vi "FPGANic-Tester.vi"() -> ()   [LabVIEW 2017]
uses:
  Source.Machine.Settings.ctl
  FPGANic.Events.ctl
  <vilib>/FPGAPlugInAG/PXIe-6592R/niLvFpga_Open_PXIe-6592R.vi
  <vilib>/rvi/interface/common/dynamic/niFpgaDynamicAddResources.vi
  FPGANic.Globals.vi
  <vilib>/Utility/error.llb/Error Cluster From Error Code.vi
  <vilib>/rvi/errors/niLvFpgaAdjustHostInterfaceError.vi
  <vilib>/FPGAPlugInAG/Dynamic/niLvFpga_Close_Dynamic.vi
  <vilib>/rvi/interface/nirviOpenFPGA/nirviOpenFPGA.xnode
  FPGA Bitfiles/FPGANic-Top.lvbitx
  <vilib>/rvi/interface/nirviMethod/nirviMethod.xnode
  <vilib>/rvi/interface/nirviReadWriteControl/nirviReadWriteControl.xnode
  <vilib>/rvi/interface/nirviCloseFPGA/nirviCloseFPGA.xnode
  <vilib>/FPGAPlugInAG/Dynamic/niLvFpga_ReadFifo_Dynamic.vi
  <vilib>/rvi/errors/niLvFpgaMergeErrorWithErrorCode.vi
  <vilib>/FPGAPlugInAG/Dynamic/niLvFpga_WriteFifo_Dynamic.vi
  NiFpgaLv.dll
  <vilib>/rvi/interface/Simulation/niFpgaSimulationCallBeginRW.vi
panel:
  in  "Read Probes":bool
  in  "Read Debug FIFOs":bool
  in  "Tab Control":T1(tab)
  in  "Ethernet II Params":T2={"Destination MAC"=[0, 2, 201, 85, 8, 68], "Source MAC"=[0, 1, 2, 3, 4, 5], "EtherType"=2048} {"Destination MAC" format="%.0x"; "Source MAC" format="%.02x"; "EtherType" format="%.0x"}
  in  "IPv4 Params":T3={"Destination IP"=[10, 0, 1, 100], "Source IP"=[10, 0, 1, 101], "Protocol"=17}
  in  "UDP Params":T4={"Source Port"=35312, "Destination Port"=35312, "Payload"="ABCD"}
  in  "MAC & IP":T5={"MAC Address"=[0, 1, 2, 3, 4, 5], "IP Address"=[10, 0, 1, 101]} {"MAC Address" format="%.0x"}
  out "Write Probe 2":u64[](array[numeric]) format="%.0x"
  out "Write Probe 1":u64[](array[numeric]) format="%.0x"
  out "Read Probe":u64[](array[numeric]) format="%.0x"
  out "Debug FIFO 2":u32[](array[numeric]) format="%.0x"
  out "Debug FIFO 1":u32[](array[numeric]) format="%.0x"
  out "UDP Payload":u8[](array[numeric]) format="%.0x"
  in  "Clear Debug FIFOS?":bool=TRUE
  in  "AXI_STR_RXD_3_tkeep":u8=15
  out "GPIO #1 out":u32 format="%.0x"
  in  "GPIO #2 in":u32 format="%.0x"
  in  "GPIO #1 in":u32=4 format="%.0x"
  out "GPIO #2 out":u32
  out "sPort0_Power_Good":bool
  out "signal_detect_Port0":bool
  out "aBlockLockPort0":bool
  in  "Read/Write GPIO":bool
  out "error out":errorcluster
  out "Status":string
  in  "error in":errorcluster
  in  "Exit":bool
  in  "Transmit Packet":bool
  in  "Read Packet":bool
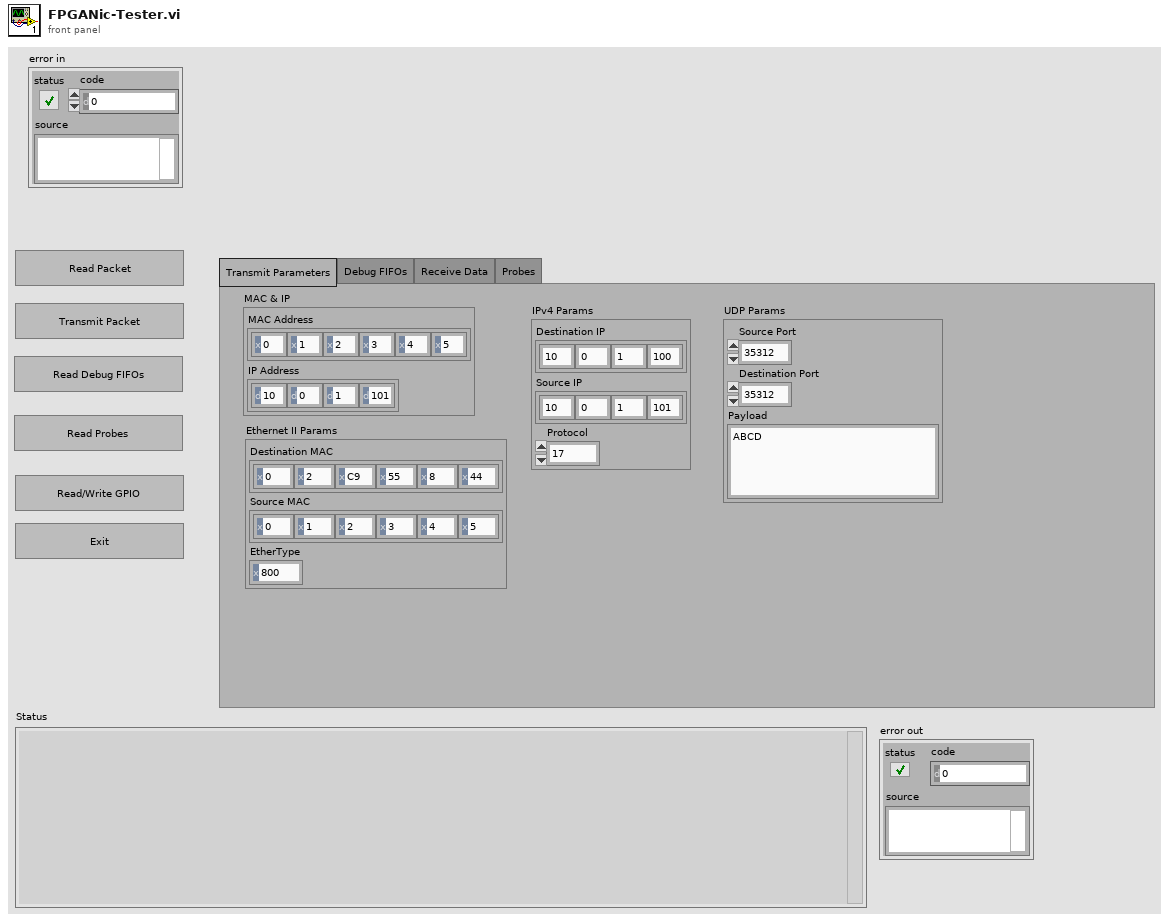
[diagram p1: front panel]
types:
  T1 = enum32{"Transmit Parameters", "Debug FIFOs", "Receive Data", "Probes"}
  T2 = cluster{"Destination MAC":u8[], "Source MAC":u8[], "EtherType":u16}
  T3 = cluster{"Destination IP":u8[], "Source IP":u8[], "Protocol":u8}
  T4 = cluster{"Source Port":u16, "Destination Port":u16, "Payload":string}
  T5 = typedef "Source.Machine.Settings.ctl" = cluster{"MAC Address":u8[], "IP Address":u8[]}
  T6 = typedef "FPGANic.Events.ctl" = enum16{"Open FPGA", "Close FPGA", "Reset UI", "Read Packet", "Transmit Packet", "Read Debug FIFOs", "Read Probes", "Read/Write GPIO"}
  T7 = cluster{"Read Probe":u64[], "Write Probe 1":u64[], "Write Probe 2":u64[], "Debug FIFO 1":u32[], "Debug FIFO 2":u32[]}
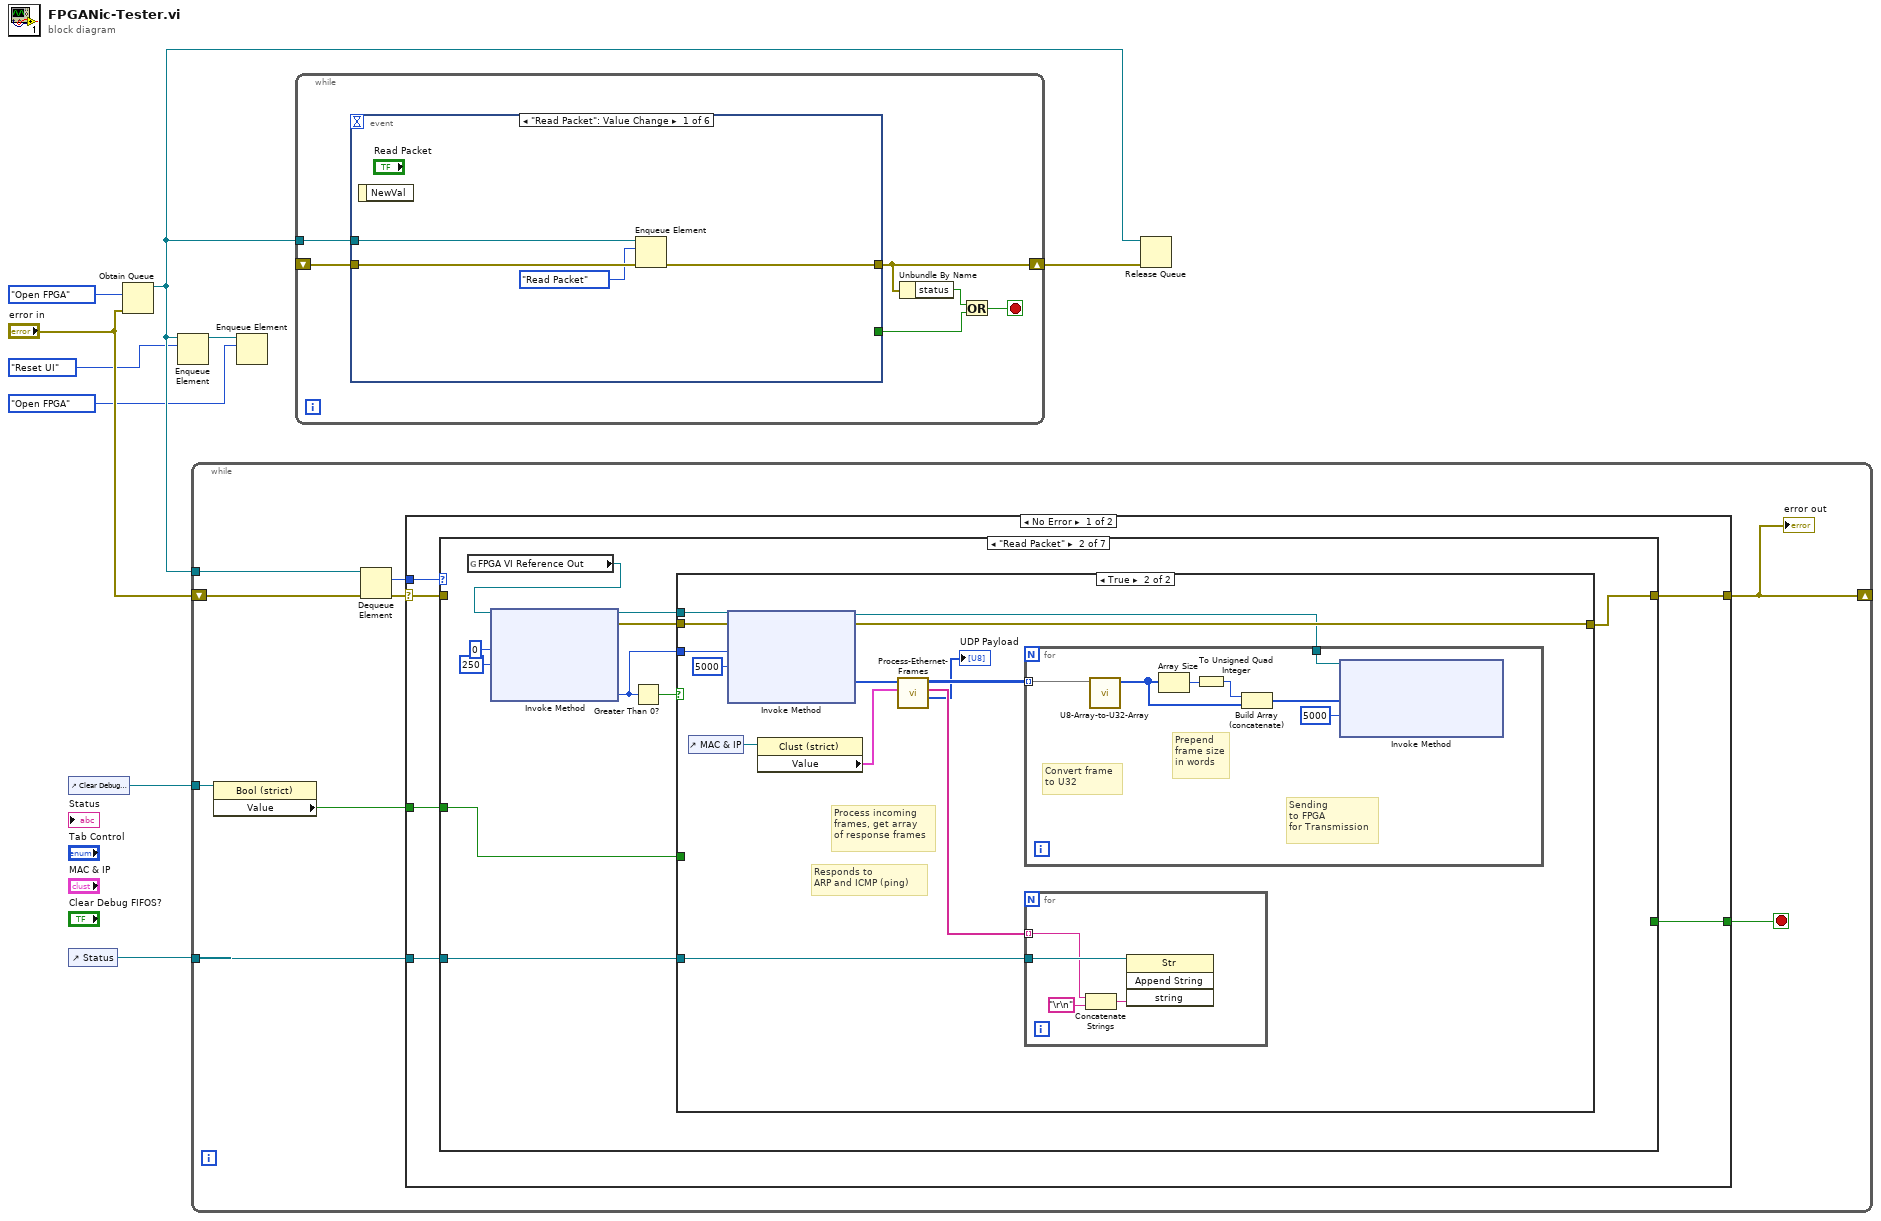
[diagram p0: block diagram]
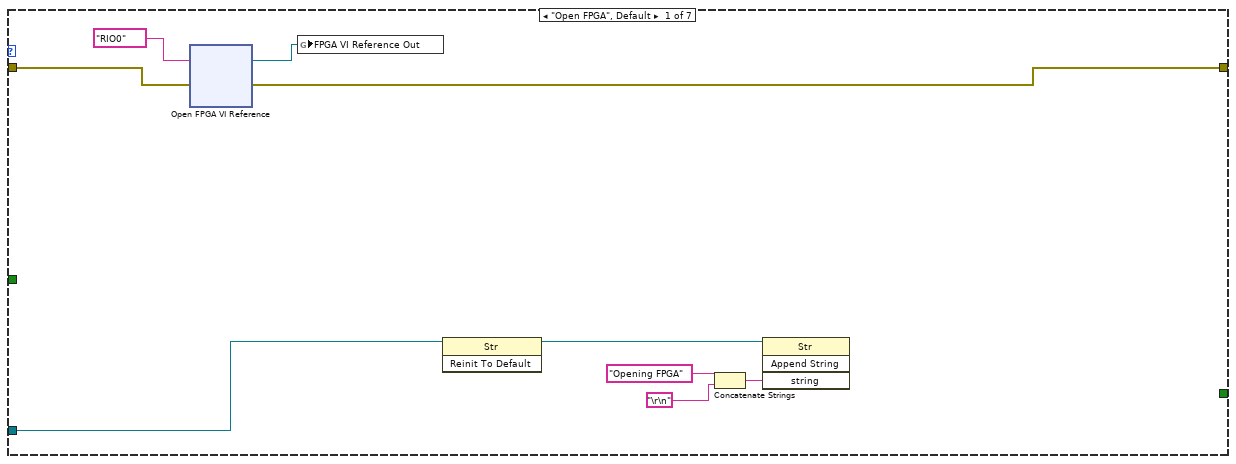
[diagram p2: hidden frame]
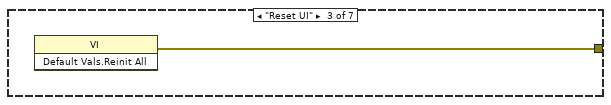
[diagram p4: hidden frame]
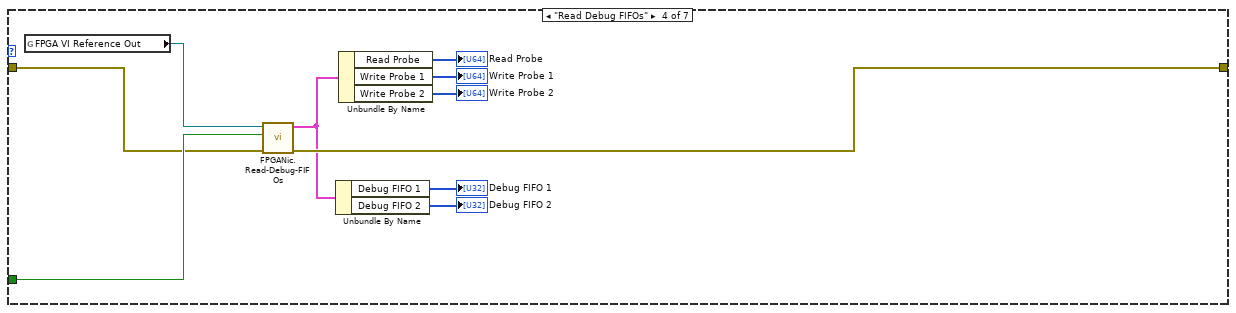
[diagram p5: hidden frame]
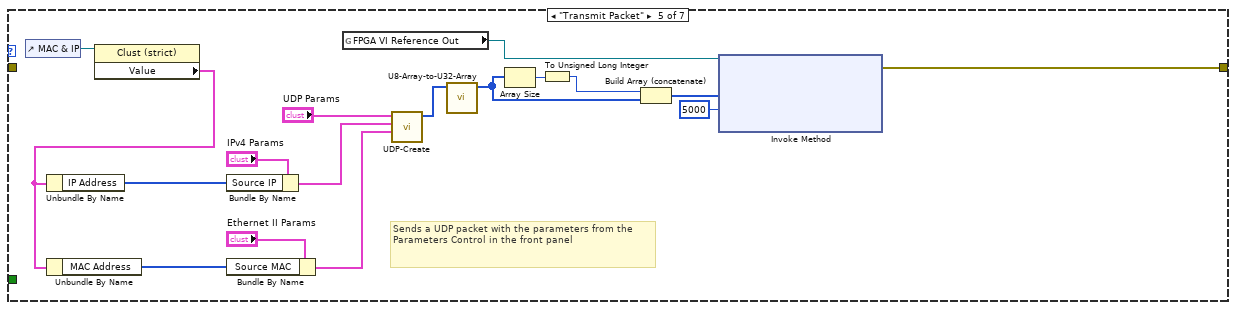
[diagram p6: hidden frame]
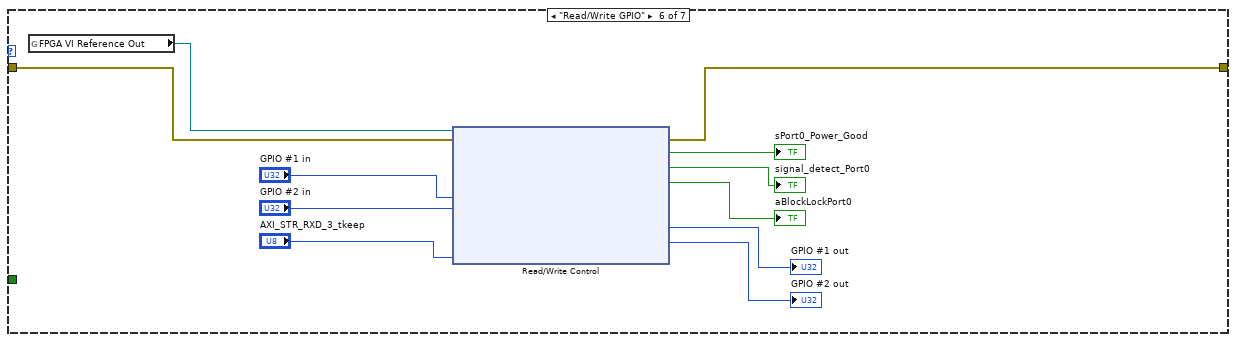
[diagram p7: hidden frame]
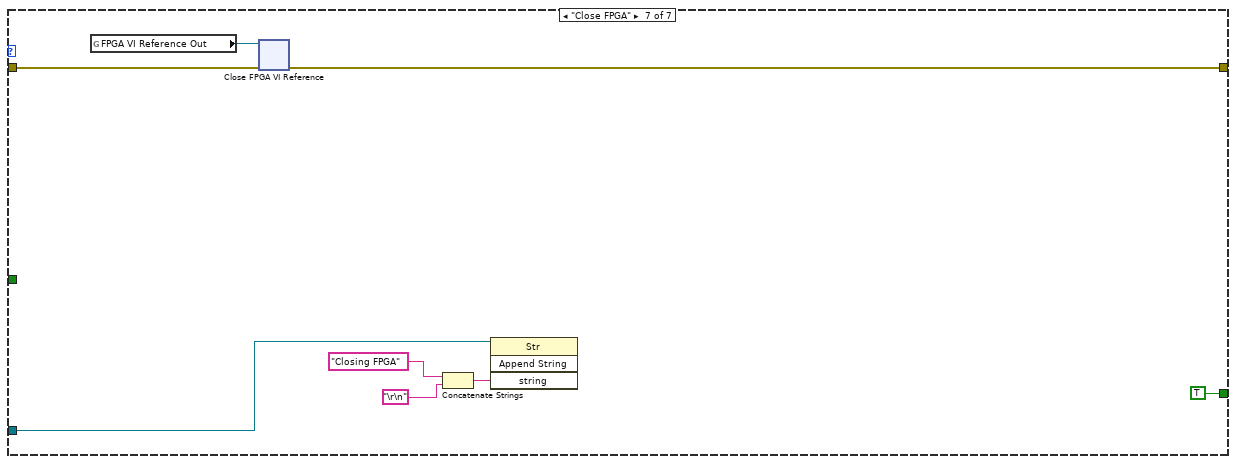
[diagram p8: hidden frame]
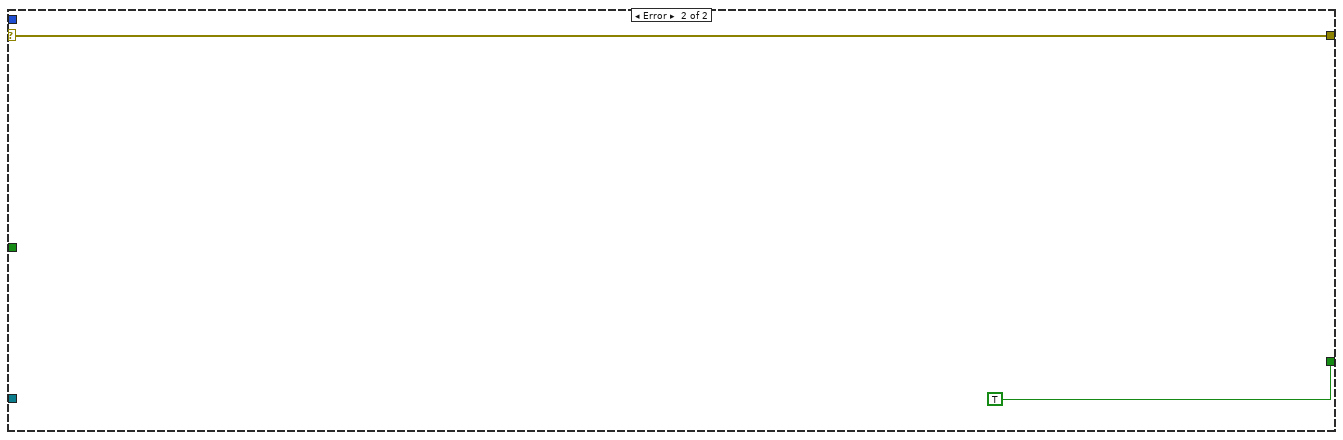
[diagram p9: hidden frame]
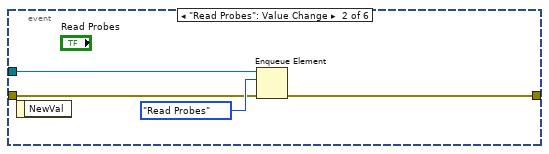
[diagram p10: hidden frame]
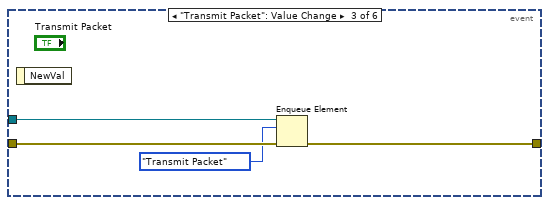
[diagram p11: hidden frame]
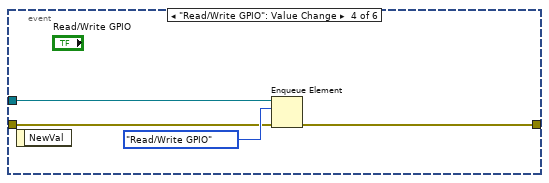
[diagram p12: hidden frame]
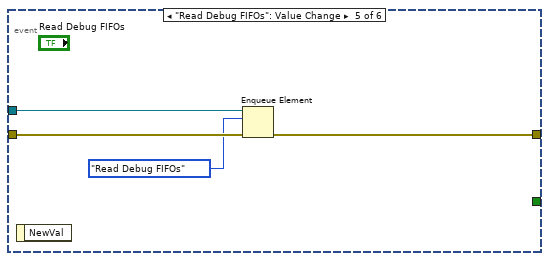
[diagram p13: hidden frame]
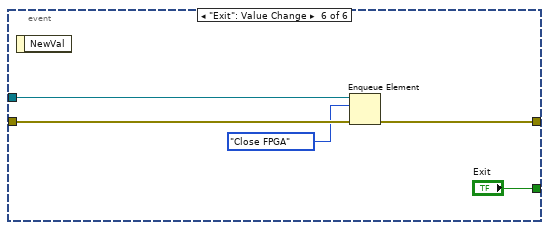
[diagram p14: hidden frame]
diagram:
  n1 = control-ref of="Clear Debug FIFOS?"() -> (w4:refnum<vi>)
  n2 = control-ref of="Status"() -> (w5:refnum<vi>)
  n3 = Obtain Queue(element data type=FPGANic.Events."Open FPGA" ("Enum"), error in (no error)="error in") -> (queue out=w7:refnum<queue>)  [unwired: 3 in, 2 out]
  n4 = Enqueue Element(queue=w7, element=FPGANic.Events."Reset UI" ("Enum")) -> (queue out=w3:refnum<queue>)  [unwired: 2 in, 2 out]
  n5 = while {
    tunnel: w7 -> [w18]
    shift-right: [w13] -> _
    shift-left: "error in" -> [w14]
    tunnel: w5 -> [w12]
    tunnel: w4 -> [w11]
    stop <- w15 stop-if-true
    n6 = property class="Bool (strict)"(reference=w11) -> ("Value"=w10:bool)  [unwired: 1 in, 2 out]
    n7 = Dequeue Element(queue=w18, error in (no error)=w14) -> (element=w16:T6, error out=w17:errorcluster)  [unwired: 1 in, 2 out]
    n8 = case shown="No Error" w17 {
      selector: w17 -> [w19 w116]
      tunnel: w16 -> [w24 _]
      tunnel: [w23 TRUE] -> w15
      tunnel: [w22 w116] -> w13
      tunnel: w12 -> [w21 _]
      tunnel: w10 -> [w20 _]
      frame No Error {
        n9 = case shown="\"Read Packet\"" w24 {
          tunnel: [_ _ _ _ _ _ TRUE] -> w23
          tunnel: [w33 w38 w69 w77 w94 w99 w114] -> w22
          tunnel: w21 -> [w29 w34 _ _ _ _ w110]
          tunnel: w20 -> [_ w36 _ w78 _ _ _]
          tunnel: w19 -> [w26 _ _ w76 _ w97 w108]
          frame "Open FPGA", Default {
            n10 = xnode "Open FPGA VI Reference"("error in"=w26, "resource name"=tag "RIO0") -> ("FPGA VI Reference Out"=w25:refnum<k20>, "error out"=w33:errorcluster)
            n11 = global write "FPGANic.Globals.vi" "FPGA VI Reference Out"(w25) -> ()
            n12 = invoke class="Str" method="Reinit To Default"(reference=w29) -> (reference out=w28:refnum<vi>)  [unwired: 2 in, 2 out]
            n13 = Concatenate Strings("Opening FPGA" ("string"), "\r\n") -> (w32:string)
            n14 = invoke class="Str" method="Append String"(reference=w28, "string"=w32) -> ()  [unwired: 2 in, 4 out]
          }
          frame "Read Packet" {
            n15 = global read "FPGANic.Globals.vi" "FPGA VI Reference Out"() -> (w35:refnum<k20>)
            n16 = xnode "Invoke Method"("FPGA VI Reference In"=w35, "Number of Elements"=u32 0, "Timeout (ms)"=250) -> ("FPGA VI Reference Out"=w40:refnum<k20>, "error out"=w39:errorcluster, "Elements Remaining"=w37:u32)  [unwired: 1 in, 1 out]
            n17 = Greater Than 0?(x=w37) -> (x > 0?=w41:bool)
            n18 = case shown="True" w41 {
              tunnel: w40 -> [_ w56]
              tunnel: w39 -> [w44 w55]
              tunnel: [w44 w53] -> w38
              tunnel: w37 -> [_ w54]
              tunnel: w36 -> [_ _]
              tunnel: w34 -> [_ w47]
              frame False {
              }
              frame True {
                # "Responds to\nARP and ICMP (ping)"
                # "Process incoming\nframes, get array\nof response frames"
                n19 = control-ref of="MAC & IP"() -> (w50:refnum<vi>)
                n20 = xnode "Invoke Method"("FPGA VI Reference In"=w56, "error in"=w55, "Number of Elements"=w54, "Timeout (ms)"=5000) -> ("FPGA VI Reference Out"=w48:refnum<k20>, "error out"=w53:errorcluster, "Data"=w52:u64[])  [unwired: 1 out]
                n21 = property class="Clust (strict)"(reference=w50) -> ("Value"=w49:T5)  [unwired: 1 in, 2 out]
                n22 = call "Process-Ethernet-Frames.vi"("Source Machine\nSettings"=w49, "Raw Data\nStream"=w52) -> ("UDP Payload"=→"UDP Payload":u8[], "Messages"=w46:string[], "Frames to send"=w51:u8[][])  [unwired: 7 in]
                n23 = for {
                  tunnel: w51 -> [w68] mode=indexing
                  tunnel: w48 -> [w62]
                  # "Prepend\nframe size\nin words"
                  # "Sending\nto FPGA\nfor Transmission"
                  # "Convert frame\nto U32"
                  n24 = call "U8-Array-to-U32-Array.vi"("Frame U8[] in"=w68) -> ("Frame U32[] out"=w63:u32[])  [unwired: 10 in]
                  n25 = Array Size(array=w63) -> (size(s)=w67:i32)
                  n26 = To Unsigned Quad Integer(1:w67) -> (0:w66:u64)
                  n27 = Build Array (concatenate)(w66, w63) -> (w65:u64[])
                  n28 = xnode "Invoke Method"("FPGA VI Reference In"=w62, "Data"=w65, "Timeout (ms)"=5000) -> ()  [unwired: 1 in, 3 out]
                }
                n29 = for {
                  tunnel: w47 -> [w59]
                  tunnel: w46 -> [w58] mode=indexing
                  n30 = Concatenate Strings(w58, "\r\n") -> (w61:string)
                  n31 = invoke class="Str" method="Append String"(reference=w59, "string"=w61) -> ()  [unwired: 2 in, 4 out]
                }
              }
            }
          }
          frame "Reset UI" {
            n32 = invoke class="VI" method="Default Vals.Reinit All"() -> (error out=w69:errorcluster)  [unwired: 3 in, 2 out]
          }
          frame "Read Debug FIFOs" {
            n33 = global read "FPGANic.Globals.vi" "FPGA VI Reference Out"() -> (w79:refnum<k20>)
            n34 = call "FPGANic.Read-Debug-FIFOs.vi"("error in"=w76, "Value"=w78, "FPGA VI Reference Out"=w79) -> ("error out"=w77:errorcluster, "Debug Data"=w72:T7)  [unwired: 7 in]
            n35 = Unbundle By Name(w72) -> ("Debug FIFO 1"=→"Debug FIFO 1":u32[], "Debug FIFO 2"=→"Debug FIFO 2":u32[])
            n36 = Unbundle By Name(w72) -> ("Read Probe"=→"Read Probe":u64[], "Write Probe 1"=→"Write Probe 1":u64[], "Write Probe 2"=→"Write Probe 2":u64[])
          }
          frame "Transmit Packet" {
            # "Sends a UDP packet with the parameters from the\nParameters Control in the front panel"
            n37 = control-ref of="MAC & IP"() -> (w83:refnum<vi>)
            n38 = property class="Clust (strict)"(reference=w83) -> ("Value"=w81:T5)  [unwired: 1 in, 2 out]
            n39 = Unbundle By Name(w81) -> ("IP Address"=w82:u8[])
            n40 = Unbundle By Name(w81) -> ("MAC Address"=w80:u8[])
            n41 = Bundle By Name(cluster="IPv4 Params", "Source IP"=w82) -> (w84:T3)
            n42 = Bundle By Name(cluster="Ethernet II Params", "Source MAC"=w80) -> (w85:T2)
            n43 = global read "FPGANic.Globals.vi" "FPGA VI Reference Out"() -> (w93:refnum<k20>)
            n44 = call "UDP-Create.vi"("Ethernet II Params"=w85, "IPv4 Params"=w84, "UDP Params"="UDP Params") -> ("Ethernet Frame"=w92:u8[])  [unwired: 6 in, 2 out]
            n45 = call "U8-Array-to-U32-Array.vi"("Frame U8[] in"=w92) -> ("Frame U32[] out"=w89:u32[])  [unwired: 10 in]
            n46 = Array Size(array=w89) -> (size(s)=w91:i32)
            n47 = To Unsigned Long Integer(number=w91) -> (unsigned 32bit integer=w90:u32)
            n48 = Build Array (concatenate)(w90, w89) -> (w88:u32[])
            n49 = xnode "Invoke Method"("FPGA VI Reference In"=w93, "Data"=w88, "Timeout (ms)"=5000) -> ("error out"=w94:errorcluster)  [unwired: 1 in, 2 out]
          }
          frame "Read/Write GPIO" {
            n50 = global read "FPGANic.Globals.vi" "FPGA VI Reference Out"() -> (w98:refnum<k20>)
            n51 = xnode "Read/Write Control"("FPGA VI Reference In"=w98, "error in"=w97, "GPIO #1 in"="GPIO #1 in", "GPIO #2 in"="GPIO #2 in", "d_microblaze_i\\AXI_STR_RXD_3_tkeep"="AXI_STR_RXD_3_tkeep") -> ("error out"=w99:errorcluster, "sPort0_Power_Good"=→"sPort0_Power_Good":bool, "signal_detect_Port0"=→"signal_detect_Port0":bool, "aBlockLockPort0"=→"aBlockLockPort0":bool, "GPIO #1 out"=→"GPIO #1 out":u32, "GPIO #2 out"=→"GPIO #2 out":u32)  [unwired: 1 out]
          }
          frame "Close FPGA" {
            n52 = global read "FPGANic.Globals.vi" "FPGA VI Reference Out"() -> (w109:refnum<k20>)
            n53 = xnode "Close FPGA VI Reference"("FPGA VI Reference In"=w109, "error in"=w108) -> ("error out"=w114:errorcluster)
            n54 = Concatenate Strings("Closing FPGA" ("string"), "\r\n") -> (w113:string)
            n55 = invoke class="Str" method="Append String"(reference=w110, "string"=w113) -> ()  [unwired: 2 in, 4 out]
          }
        }
      }
      frame Error {
      }
    }
    "error out" <- w13
  }
  n56 = Enqueue Element(queue=w3, element=FPGANic.Events."Open FPGA" ("Enum")) -> ()  [unwired: 2 in, 3 out]
  n57 = while {
    tunnel: w7 -> [w123]
    shift-right: [w118] -> w8
    shift-left: _ -> [w119]
    stop <- w121 stop-if-true
    n58 = event shown="[0] \"Read Packet\": Value Change" {
      selector: _ -> [_ _ _ _ _ _]
      dyn-events: _ -> [_ _ _ _ _ _]
      timeout: _ -> [_ _ _ _ _ _]
      tunnel: w123 -> [w127 w128 w135 w138 w143 w148]
      tunnel: [w126 w129 w133 w136 w140 w147] -> w118
      tunnel: [_ _ _ _ _ "Exit"] -> w120
      tunnel: w119 -> [w125 w130 w134 w137 w142 w145]
      event "Read Packet": Value Change {
        n59 = event-data() -> ()  [unwired: 1 in, 1 out]
        n60 = Enqueue Element(queue=w127, element=FPGANic.Events."Read Packet" ("Enum"), error in (no error)=w125) -> (error out=w126:errorcluster)  [unwired: 1 in, 2 out]
      }
      event "Read Probes": Value Change {
        n61 = event-data() -> ()  [unwired: 1 in, 1 out]
        n62 = Enqueue Element(queue=w128, element=FPGANic.Events."Read Probes" ("Enum"), error in (no error)=w130) -> (error out=w129:errorcluster)  [unwired: 1 in, 2 out]
      }
      event "Transmit Packet": Value Change {
        n63 = event-data() -> ()  [unwired: 1 in, 1 out]
        n64 = Enqueue Element(queue=w135, element=FPGANic.Events."Transmit Packet" ("Enum"), error in (no error)=w134) -> (error out=w133:errorcluster)  [unwired: 1 in, 2 out]
      }
      event "Read/Write GPIO": Value Change {
        n65 = event-data() -> ()  [unwired: 1 in, 1 out]
        n66 = Enqueue Element(queue=w138, element=FPGANic.Events."Read/Write GPIO" ("Enum"), error in (no error)=w137) -> (error out=w136:errorcluster)  [unwired: 1 in, 2 out]
      }
      event "Read Debug FIFOs": Value Change {
        n67 = event-data() -> ()  [unwired: 1 in, 1 out]
        n68 = Enqueue Element(queue=w143, element=FPGANic.Events."Read Debug FIFOs" ("Enum"), error in (no error)=w142) -> (error out=w140:errorcluster)  [unwired: 1 in, 2 out]
      }
      event "Exit": Value Change {
        n69 = event-data() -> ()  [unwired: 1 in, 1 out]
        n70 = Enqueue Element(queue=w148, element=FPGANic.Events."Close FPGA" ("Enum"), error in (no error)=w145) -> (error out=w147:errorcluster)  [unwired: 1 in, 2 out]
      }
    }
    n71 = Unbundle By Name(w118) -> ("status"=w122:bool)
    n72 = Or(x=w122, y=w120) -> (x .or. y?=w121:bool)
  }
  n73 = Release Queue(queue=w7, error in (no error)=w8) -> ()  [unwired: 1 in, 3 out]
